vi "enqueueElement.vi"(10 "element":string, 11 "queue":string) -> ()   [LabVIEW 2011]
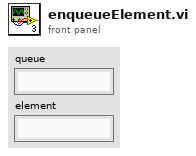
[diagram p1: front panel]
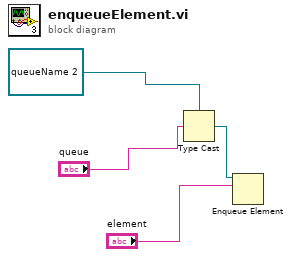
[diagram p0: block diagram]
diagram:
  n1 = Type Cast(type=refnum<queue> refnum ("队列输出"), x="queue") -> (*(type *) &x=w1:refnum<queue>)
  n2 = Enqueue Element(queue=w1, element="element") -> ()  [unwired: 2 in, 3 out]
